vi "SWEEP_CONT.vi"(0 "Session In":refnum<visa-resource-name>="GPIB0::16::INSTR", 2 "OPC?":bool, 5 "ON/OFF":u16(ring) items=["OFF", "ON"], 11 "error in":errorcluster {"code" format="%.0x"}, 12 "Timeout":u32=3000, 13 "RO (T)":bool) -> (4 "Session Out":refnum<visa-resource-name>, 8 "Read":string, 15 "error out":errorcluster {"code" format="%.0x"})   [LabVIEW 2018]
doc: "Launches the Instrument I/O Assistant, which you can use to communicate with message-based instruments and graphically parse the response. For example you can communicate with an instrument that uses a serial, Ethernet, or GPIB interface."
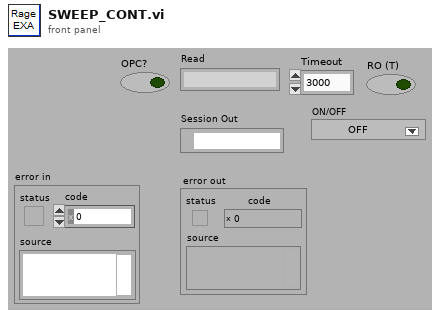
[diagram p1: front panel]
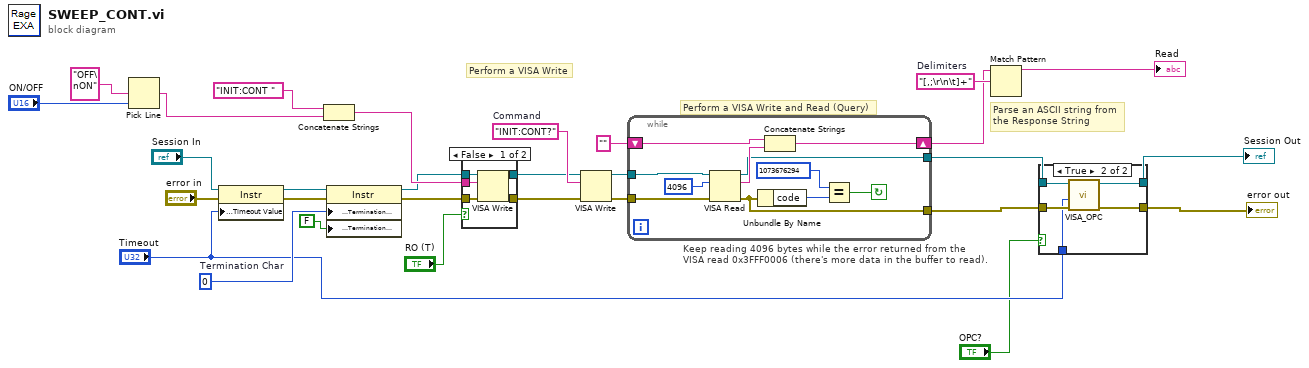
[diagram p0: block diagram]
diagram:
  w13 = "[,;\r\n\t]+"  # Delimiters
  w15 = "INIT:CONT?"  # Command
  w25 = u8 0  # Termination Char
  # "Parse an ASCII string from the Response String"
  # "Perform a VISA Write and Read (Query)"
  # "Keep reading 4096 bytes while the error returned from the\nVISA read 0x3FFF0006 (there's more data in the buffer to read)."
  # "Perform a VISA Write"
  n1 = Pick Line(multi-line string="OFF\nON", line index="ON/OFF") -> (output string=w1:string)  [unwired: 1 in]
  n2 = property class="Instr"(reference="Session In", error in="error in", "General Settings:Timeout Value"="Timeout") -> (reference out=w24:refnum<visa-resource-name>, error out=w27:errorcluster)
  n3 = Concatenate Strings("INIT:CONT " ("staticText"), w1) -> (w20:string)
  n4 = property class="Instr"(reference=w24, error in=w27, "Message Based Settings:Termination Character"=w25, "Message Based Settings:Termination Character Enable"=FALSE ("enable")) -> (reference out=w11:refnum<visa-resource-name>, error out=w26:errorcluster)
  n5 = case shown="False" "RO (T)" {
    tunnel: w26 -> [w34 w35]
    tunnel: [w33 w35] -> w21
    tunnel: w20 -> [w32 _]
    tunnel: w11 -> [w31 w36]
    tunnel: [w30 w36] -> w10
    frame False {
      n6 = VISA Write(VISA resource name=w31, write buffer=w32, error in (no error)=w34) -> (VISA resource name out=w30:refnum<visa-resource-name>, error out=w33:errorcluster)  [unwired: 1 out]
    }
    frame True {
    }
  }
  n7 = VISA Write(VISA resource name=w10, write buffer=w15, error in (no error)=w21) -> (VISA resource name out=w19:refnum<visa-resource-name>, error out=w18:errorcluster)  [unwired: 1 out]
  n8 = while {
    tunnel: w19 -> [w44]
    shift-right: [w38] -> w12
    shift-left: "" -> [w43]
    tunnel: w18 -> [w41]
    tunnel: [w40] -> w17
    tunnel: [w37] -> w7
    stop <- w39 continue-if-true
    n9 = VISA Read(VISA resource name=w44, byte count=u32 4096 ("byte count (0)"), error in (no error)=w41) -> (VISA resource name out=w37:refnum<visa-resource-name>, read buffer=w42:string, error out=w40:errorcluster)  [unwired: 1 out]
    n10 = Unbundle By Name(w40) -> ("code"=w46:i32)
    n11 = Concatenate Strings(w43, w42) -> (w38:string)
    n12 = Equal?(x=1073676294, y=w46) -> (x = y?=w39:bool)
  }
  n13 = Match Pattern(string=w12, regular expression=w13) -> (before substring=→"Read":string)  [unwired: 4 out]
  n14 = case shown="True" "OPC?" {
    tunnel: w17 -> [w48 w54]
    tunnel: [w48 w53] -> w8
    tunnel: w7 -> [w49 w52]
    tunnel: [w49 w51] -> w6
    tunnel: "Timeout" -> [_ w50]
    frame False {
    }
    frame True {
      n15 = call "VISA_OPC.vi"("error in"=w54, "Timeout"=w50, "Session In"=w52) -> ("error out"=w53:errorcluster, "Session Out"=w51:refnum<visa-resource-name>)  [unwired: 6 in, 1 out]
    }
  }
  "error out" <- w8
  "Session Out" <- w6
